vi "IR Cam Exit_SD.vi"   [LabVIEW 2015]
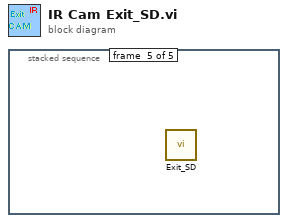
[diagram p0: block diagram]
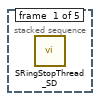
[diagram p2: hidden frame]
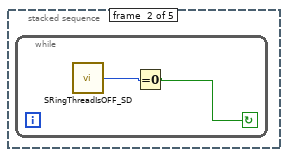
[diagram p3: hidden frame]
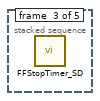
[diagram p4: hidden frame]
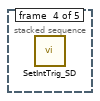
[diagram p5: hidden frame]
diagram:
  n1 = stacked-sequence {
    frame #0 {
      n2 = call "SRingStopThread_SD.vi"() -> ()  [unwired: 1 in]
    }
    frame #1 {
      n3 = while {
        stop <- w1 continue-if-true
        n4 = call "SRingThreadIsOFF_SD.vi"() -> ("ThreadIsOFF"=w2:u8)
        n5 = Equal To 0?(x=w2) -> (x = 0?=w1:bool)
      }
    }
    frame #2 {
      n6 = call "FFStopTimer_SD.vi"() -> ()  [unwired: 1 in]
    }
    frame #3 {
      n7 = call "SetIntTrig_SD.vi"() -> ()  [unwired: 1 in]
    }
    frame #4 {
      n8 = call "Exit_SD.vi"() -> ()  [unwired: 1 in]
    }
  }
